vi "Save File Folder Dates.vi"(8 "Error In":errorcluster) -> (0 "Error Out":errorcluster, 1 "Year/Month/Day":string, 2 "Year/Month":string, 3 "Year":string)   [LabVIEW 2018, in "Save File.lvlib"]
uses:
  Save File.lvlib
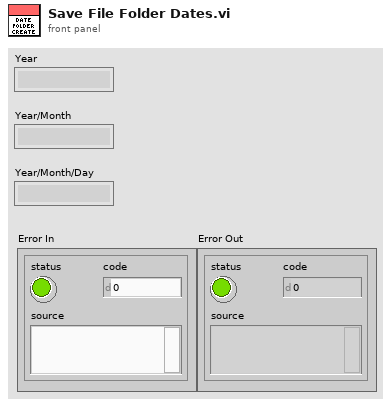
[diagram p1: front panel]
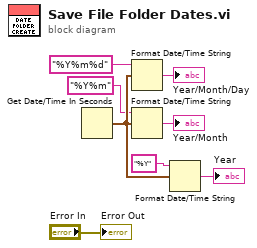
[diagram p0: block diagram]
diagram:
  n1 = Get Date/Time In Seconds() -> (seconds since 1Jan1904=w4:timestamp)
  n2 = Format Date/Time String(time format string (%c)="%Y%m%d", seconds (now)=w4) -> (date/time string=→"Year/Month/Day":string)  [unwired: 1 in]
  n3 = Format Date/Time String(time format string (%c)="%Y%m", seconds (now)=w4) -> (date/time string=→"Year/Month":string)  [unwired: 1 in]
  n4 = Format Date/Time String(time format string (%c)="%Y", seconds (now)=w4) -> (date/time string=→"Year":string)  [unwired: 1 in]
  "Error Out" <- "Error In"
